vi "gettheta.vi"() -> (3 "function return":dbl)   [LabVIEW 2019, in "HapticSTM.lvlib"]
doc: "extern \"C\" __declspec(dllexport) double gettheta();"
uses:
  HapticSTM.lvlib
  <userlib>/HapticSTM/HapticSTM.dll
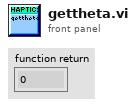
[diagram p1: front panel]
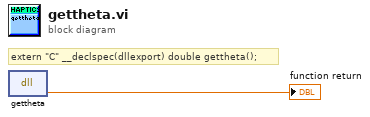
[diagram p0: block diagram]
diagram:
  # "extern \"C\" __declspec(dllexport) double gettheta();"
  n1 = dll-call lib="C:/Program Files/National Instruments/LabVIEW 2019/user.lib/HapticSTM/HapticSTM.*" fn="gettheta"() -> (→"function return":dbl)  [unwired: 3 in, 2 out]
